vi "Transmitter_Monokrom_Fix.vi"() -> ()   [LabVIEW 2018]
uses:
  <vilib>/picture/picture.llb/imagedata.ctl
  <instrlib>/niUSRP/niUSRP Write Tx Data (CDB Cluster).vi
panel:
  in  "Python version":string="3.12.3"
  in  "Python File Encoder Huffman":path=path "D:/Thesis Pak Pri/huffman_encoder.py"
  out "percentage compression (%)":i32
  out "size(s) 6":i32[](array[numeric])
  out "size(s) 5":i32
  out "Array":i32[](array[numeric])
  in  "array":i32[](array[numeric])
  out "iterasi":i32
  out "hasil bagi":i32
  out "sisa bagi":i32
  out "output array":i16[](array[numeric])
  in  "bit length (set)":i32=3600
  out "output cluster 2":cluster{"t0":dbl, "dt":dbl, "Y":cdb[]}
  out "error out 2":errorcluster
  out "Frame Duration 2":dbl format="%#_6p"
  out "Waveform Graph 2":cluster{"t0":dbl, "dt":dbl, "Y":dbl[]}(graph)
  out "1-bit pixmap":bool[][](array[boolean])
  out "Input Image":picture
  out "image data":T1
  in  "path to BMP file":path=path "D:/PAKPRI_LAST/PAKPRI/boo.bmp"
  in  "Modulation parameter":T2
  out "USRP CoercedParamters":T3={"coerced IQ rate"=100000.0, "coerced carrier frequency"=100000.0, "coerced gain"=0.0} {"coerced gain" format="%#_6f"; "coerced carrier frequency" format="%#_6p"; "coerced IQ rate" format="%#_6p"}
  in  "error in (no error)":errorcluster
  in  "USRP ControledParameters":T4={"active antenna"="TX1", "gain"=0.0, "carrier frequency"=915000000.0, "IQ rate"=1000000.0} {"IQ rate" format="%#_6p"; "carrier frequency" format="%#_6p"; "gain" format="%#_6f"}
  in  "device names":refnum<k15>="192.168.10.1"
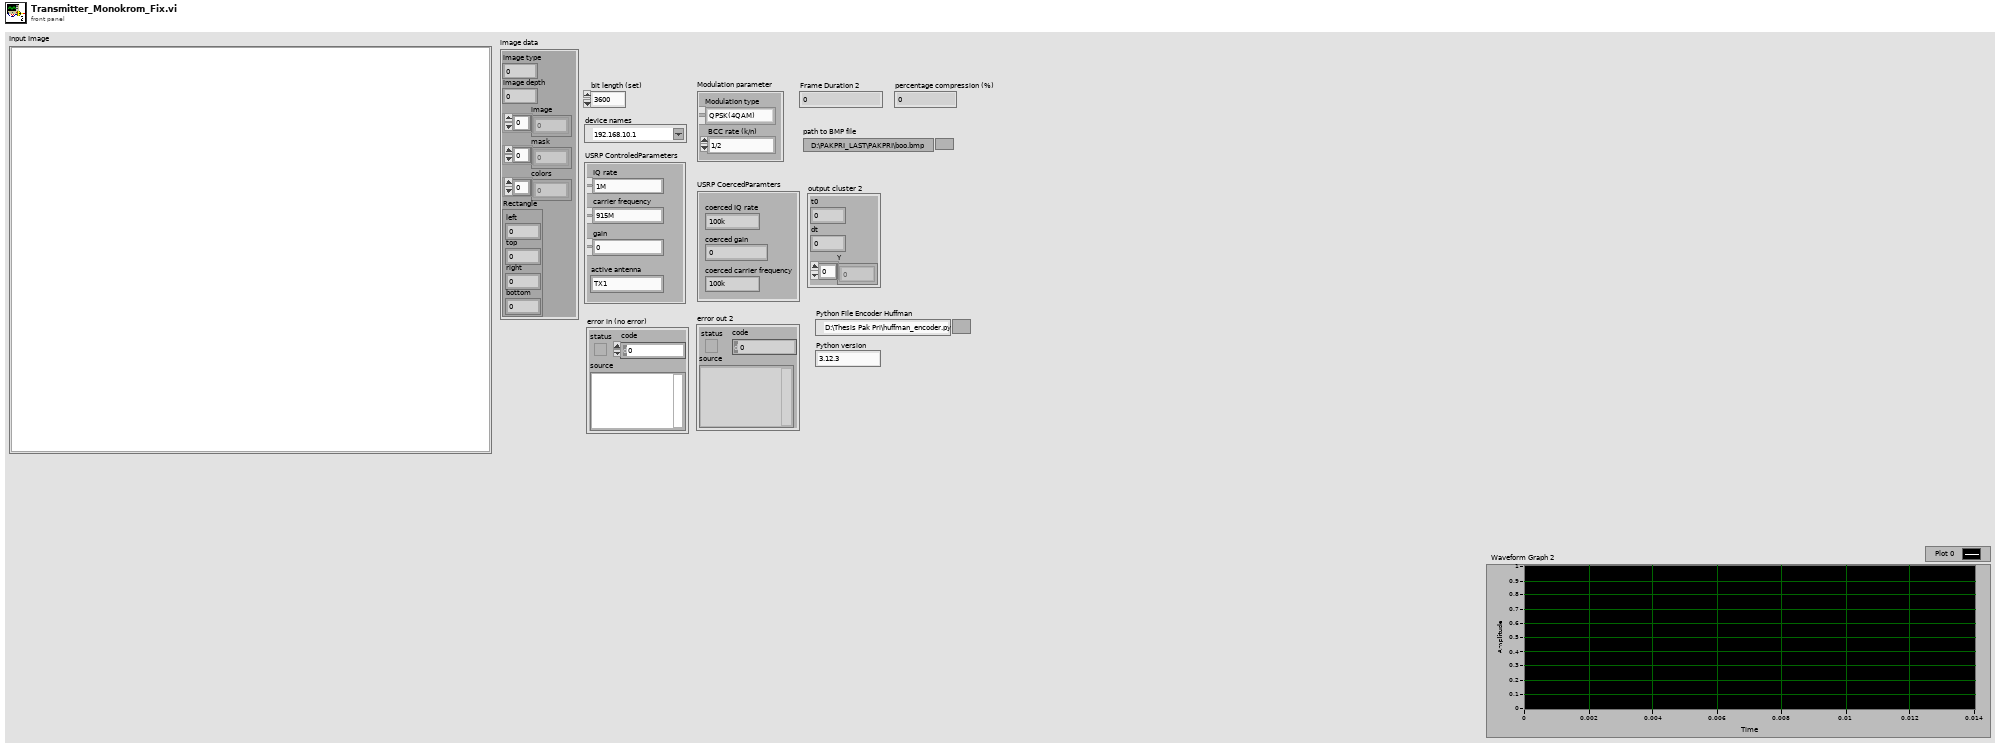
[diagram p1: front panel]
types:
  T1 = typedef "imagedata.ctl" = cluster{"image type":i32, "image depth":i32, "image":u8[], "mask":u8[], "colors":u32[], "Rectangle":cluster{"left":i16, "top":i16, "right":i16, "bottom":i16}}
  T2 = cluster{"Modulation type":enum16{"QPSK(4QAM)", "64QAM", "16QAM", "BPSK"}, "BCC rate (k/n)":enum16{"1/2", "2/3", "3/4"}}
  T3 = cluster{"coerced IQ rate":dbl, "coerced carrier frequency":dbl, "coerced gain":dbl}
  T4 = cluster{"active antenna":string, "gain":dbl, "carrier frequency":dbl, "IQ rate":dbl}
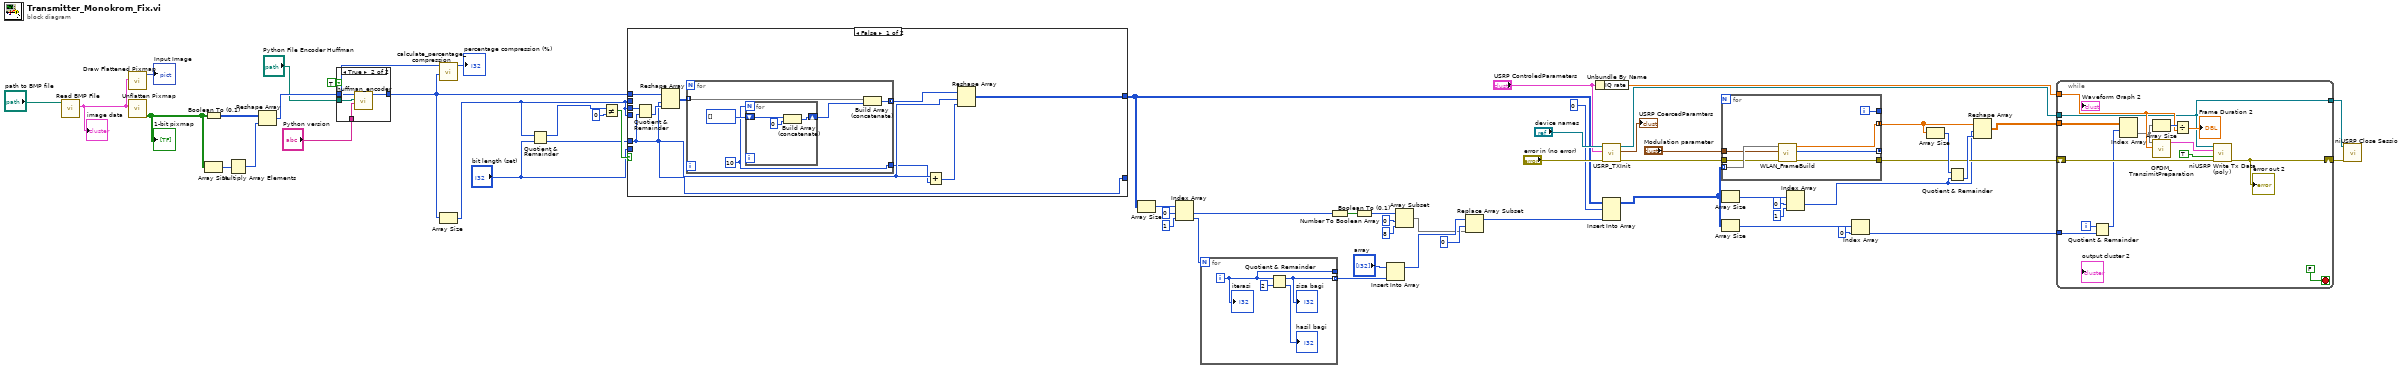
[diagram p0: block diagram]
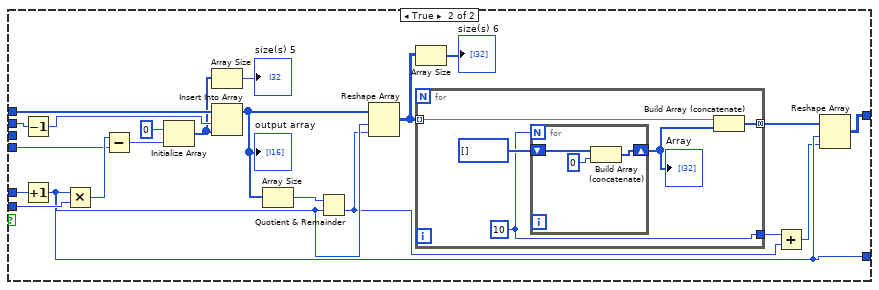
[diagram p3: hidden frame]
diagram:
  n1 = call <vilib>:"Read BMP File.vi"("path to BMP file"="path to BMP file") -> ("image data"=w53:T1)  [unwired: 8 in, 2 out]
  "image data" <- w53
  n2 = call <vilib>:"Draw Flattened Pixmap.vi"("image data"=w53) -> ("new picture"=→"Input Image":picture)  [unwired: 8 in]
  n3 = call <vilib>:"Unflatten Pixmap.vi"("image data"=w53) -> ("1-bit pixmap"=w51:bool[][])  [unwired: 4 in, 6 out]
  "1-bit pixmap" <- w51
  n4 = Boolean To (0,1)(Boolean=w51) -> (0, 1=w10:i16[][])
  n5 = Array Size(array=w51) -> (size(s)=w52:i32[])
  n6 = Multiply Array Elements(1:w52) -> (0:w50:i32)
  n7 = Reshape Array(w10, w50) -> (w9:i16[])
  n8 = case shown="True" TRUE {
    tunnel: w9 -> [w60 w64]
    tunnel: [w60 w63] -> w3
    tunnel: "Python File Encoder Huffman" -> [_ w62]
    tunnel: "Python version" -> [_ w61]
    frame False {
    }
    frame True {
      n9 = call "huffman_encoder.vi"("Python version"=w61, "module path"=w62, "bit_array"=w64) -> ("return value"=w63:i32[])  [unwired: 8 in]
    }
  }
  n10 = call "calculate_percentage_compression.vi"("compression bit length"=w3, "original bit length"=w9) -> ("percentage compression"=→"percentage compression (%)":i32)  [unwired: 9 in]
  n11 = Array Size(array=w3) -> (size(s)=w44:i32)
  n12 = Quotient & Remainder(x=w44, y="bit length (set)") -> (x-y*floor(x/y)=w49:i32, floor(x/y)=w46:i32)
  n13 = Not Equal?(x=w49, y=0) -> (x != y?=w47:bool)
  n14 = case shown="False" w47 {
    tunnel: w46 -> [w69 w102]
    tunnel: "bit length (set)" -> [_ w101]
    tunnel: w44 -> [_ w92]
    tunnel: w3 -> [w65 w98]
    tunnel: w44 -> [_ w97]
    tunnel: [w69 w90] -> _
    tunnel: [w66 w86] -> w12
    tunnel: w44 -> [w73 _]
    frame False {
      n15 = Quotient & Remainder(x=w73, y=w69) -> (floor(x/y)=w72:i32)  [unwired: 1 out]
      n16 = Reshape Array(w65, w69, w72) -> (w71:i32[][])
      n17 = for {
        tunnel: w71 -> [w77] mode=indexing
        tunnel: [w75] -> w70 mode=concatenating
        tunnel: [w74] -> w68
        w74 = 10
        n18 = for {
          N: w74 -> [_]
          shift-right: [w79] -> w76
          shift-left: i32[] [] -> [w81]
          n19 = Build Array (concatenate)(w81, 0) -> (w79:i32[])
        }
        n20 = Build Array (concatenate)(w77, w76) -> (w75:i32[])
      }
      n21 = Add(x=w69, y=w68) -> (x+y=w67:i32)
      n22 = Reshape Array(w70, w69, w67) -> (w66:i32[][])
    }
    frame True {
      n23 = Decrement(x=w97) -> (x-1=w96:i32)
      n24 = Increment(x=w102) -> (x+1=w90:i32)
      n25 = Multiply(x=w90, y=w101) -> (x*y=w93:i32)
      n26 = Subtract(x=w93, y=w92) -> (x-y=w99:i32)
      n27 = Initialize Array(0 ("element"), w99) -> (w85:i32[])
      n28 = Array Size(array=w85) -> (size(s)=→"size(s) 5":i32)
      n29 = Insert Into Array(array=w98, index=w96, new element=w85) -> (w95:i32[])
      "output array" <- w95
      n30 = Array Size(array=w95) -> (size(s)=w94:i32)
      n31 = Quotient & Remainder(x=w94, y=w90) -> (floor(x/y)=w88:i32)  [unwired: 1 out]
      n32 = Reshape Array(w95, w90, w88) -> (w82:i32[][])
      n33 = Array Size(array=w82) -> (size(s)=→"size(s) 6":i32[])
      n34 = for {
        tunnel: w82 -> [w106] mode=indexing
        tunnel: [w103] -> w91 mode=concatenating
        tunnel: [w105] -> w89
        w105 = 10
        n35 = for {
          N: w105 -> [_]
          shift-right: [w108] -> w104
          shift-left: i32[] [] -> [w110]
          n36 = Build Array (concatenate)(w110, 0) -> (w108:i32[])
        }
        "Array" <- w104
        n37 = Build Array (concatenate)(w106, w104) -> (w103:i32[])
      }
      n38 = Add(x=w89, y=w88) -> (x+y=w87:i32)
      n39 = Reshape Array(w91, w90, w87) -> (w86:i32[][])
    }
  }
  n40 = Array Size(array=w12) -> (size(s)=w24:i32[])
  n41 = Index Array(array=w24, index #1=0 ("index"), index #2=1 ("index")) -> (element #1=w20:i32, element #2=w21:i32)
  n42 = for {
    N: w21 -> [_]
    tunnel: [w112] -> _
    tunnel: [w111] -> w25 mode=indexing
    i -> [w112]
    n43 = Quotient & Remainder(x=w112, y=2) -> (x-y*floor(x/y)=w111:i32, floor(x/y)=→"hasil bagi":i32)
    "sisa bagi" <- w111
    "iterasi" <- w112
  }
  n44 = Number To Boolean Array(number=w20) -> (Boolean array=w27:bool[])
  n45 = Boolean To (0,1)(Boolean=w27) -> (0, 1=w18:i16[])
  n46 = Insert Into Array(array="array", new element=w25) -> (w15:i32[])  [unwired: 1 in]
  n47 = Array Subset(array=w18, index=0, length=8) -> (w11:i16[])
  n48 = Replace Array Subset(array=w15, new element=w11, index=0) -> (w13:i32[])
  n49 = Unbundle By Name("USRP ControledParameters") -> ("IQ rate"=w34:dbl)
  n50 = call "USRP_TXInit.vi"("device names"="device names", "USRP ControledParameters"="USRP ControledParameters", "error in (no error)"="error in (no error)") -> ("session handle out"=w33:refnum<k15>, "USRP CoercedParamters"=→"USRP CoercedParamters":T3, "error out"=w42:errorcluster)  [unwired: 5 in]
  n51 = Insert Into Array(array=w12, index (row)=0, new element=w13) -> (w4:i32[][])  [unwired: 1 in]
  n52 = for {
    tunnel: w4 -> [w121] mode=indexing
    tunnel: "Modulation parameter" -> [w119]
    tunnel: w42 -> [w118]
    tunnel: [w120] -> w31 mode=concatenating
    tunnel: [w116] -> w28
    tunnel: [w117] -> _ mode=concatenating
    tunnel: [w115] -> _
    i -> [w115]
    n53 = call "WLAN_FrameBuild.vi"("error in (no error)"=w118, "Modulation parameter"=w119, "data in"=w121) -> ("error out"=w116:errorcluster, "output bit stream 3"=w117:i8[], "output array"=w120:cdb[])  [unwired: 5 in, 1 out]
  }
  n54 = Array Size(array=w4) -> (size(s)=w41:i32[])
  n55 = Array Size(array=w4) -> (size(s)=w37:i32[])
  n56 = Index Array(array=w41, index #1=0 ("index"), index #2=1 ("index")) -> (element #1=w5:i32)  [unwired: 1 out]
  n57 = Index Array(array=w37, index=0) -> (element=w35:i32)
  n58 = Array Size(array=w31) -> (size(s)=w30:i32)
  n59 = Quotient & Remainder(x=w30, y=w5) -> (floor(x/y)=w29:i32)  [unwired: 1 out]
  n60 = Reshape Array(w31, w5, w29) -> (w6:cdb[][])
  n61 = while {
    tunnel: w6 -> [w122]
    tunnel: w34 -> [w129]
    shift-right: [w130] -> w38
    shift-left: w28 -> [w131]
    tunnel: w33 -> [w124]
    tunnel: w35 -> [w125]
    tunnel: [w124] -> w32
    i -> [w128]
    stop <- FALSE stop-if-true
    n62 = Quotient & Remainder(x=w128, y=w125) -> (x-y*floor(x/y)=w127:i32)  [unwired: 1 out]
    n63 = Index Array(array=w122, index (row)=w127) -> (element=w123:cdb[])  [unwired: 1 in]
    n64 = Array Size(array=w123) -> (size(s)=w135:i32)
    n65 = call "OFDM_TransimitPreparation.vi"("IQ rate"=w129, "array"=w123) -> ("output cluster"=w134:cluster{"t0":dbl, "dt":dbl, "Y":cdb[]})  [unwired: 8 in, 1 out]
    n66 = Divide(x=w135, y=w129) -> (x/y=→"Frame Duration 2":dbl)
    n67 = call-poly <instrlib>:"niUSRP Write Tx Data (poly).vi"("session handle"=w124, "data"=w134, "end of data?"=TRUE, "error in (no error)"=w131) -> ("error out"=w130:errorcluster)  [unwired: 10 in, 1 out]
    "error out 2" <- w130
  }
  n68 = call <instrlib>:"niUSRP Close Session.vi"("session handle"=w32, "error in (no error)"=w38) -> ()  [unwired: 13 in, 1 out]
